vi "Visa_Write read_UI GETPIN.vi"(0 "Serial Device in":refnum<class "Serial Device.lvclass">, 1 "VISA resource name":refnum<visa-resource-name>, 2 "Command to Send":string, 3 "Expected Response":string, 4 "Buttons":bool[](array[boolean]), 5 "error in (no error)":errorcluster) -> (13 "Valor pin":bool, 14 "Serial Device out":refnum<class "Serial Device.lvclass">, 15 "VISA resource name":refnum<visa-resource-name>, 16 "Response":string, 17 "Port":string, 18 "PIN":string, 19 "error out":errorcluster)   [LabVIEW 2020, in "Serial Device.lvclass"]
uses:
  Serial Device.lvclass
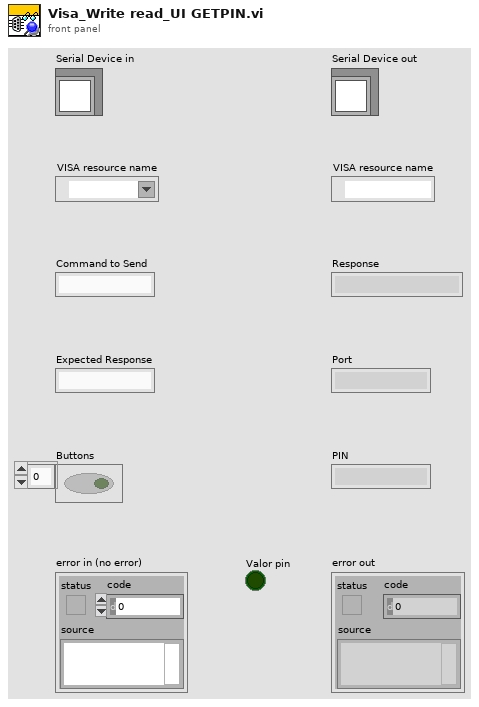
[diagram p1: front panel]
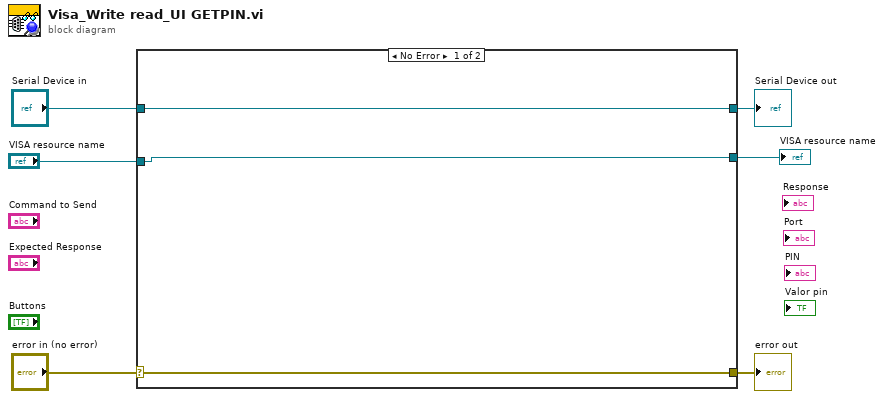
[diagram p0: block diagram]
diagram:
  n1 = case shown="No Error" "error in (no error)" {
    selector: "error in (no error)" -> [w8 w11]
    tunnel: [w8 w11] -> w5
    tunnel: [w9 w10] -> w3
    tunnel: "Serial Device in" -> [w9 w10]
    tunnel: "VISA resource name" -> [w7 _]
    tunnel: [w7 _] -> w1
    frame No Error {
    }
    frame Error {
    }
  }
  "error out" <- w5
  "Serial Device out" <- w3
  "VISA resource name" <- w1
